vi "TestPattern.vi"() -> ()   [LabVIEW 2016]
uses:
  C:/Users/Aerotech/Documents/BNLStaveAssembly-blueprint/Bin/Aerotech.A3200.dll
  BNLStaveAssembly-blueprint/Bin/Aerotech.A3200.dll
  <vilib>/Utility/file.llb/Read Delimited Spreadsheet (DBL).vi
  <vilib>/Utility/file.llb/Write Delimited Spreadsheet (DBL).vi
  <vilib>/Utility/file.llb/Write Delimited Spreadsheet (I64).vi
panel:
  out "y length":i32
  out "x length":i32
  in  "y array":path
  out "y array":dbl[](array[numeric])
  in  "path to just x array":path
  out "just x array":dbl[](array[numeric])
  out "trial 2":cluster{dbl[], dbl[]}
  in  "Lowest Z Position":dbl=38.0
  in  "XYZ Stage Control":refnum<k24>
  in  "Axis speeds (mm/s)":T1={"vX [mm]"=49.0, "vY [mm]"=49.0, "vZ [mm] "=49.0}
  out "Final Position":T2={"Final X"=-325.49379764644783, "Final Y"=23.533617154160947, "Final Z"=34.99956596392527}
  out "y coord":dbl[](array[numeric])
  out "x coord":dbl[](array[numeric])
  out "all coords":dbl[][](array[numeric])
  in  "file path (dialog if empty)":path
  in  "append to file? (new file:F)":bool
  in  "x dist":dbl=90.0
  in  "y dist":dbl=90.0
  out "Trial 1":dbl[][](array[numeric])
  out "dx":dbl
  out "dy":dbl
  in  "module lenght y":dbl=90.0
  in  "module lenght x":dbl=90.0
  out "Array":bool[][](array[boolean])
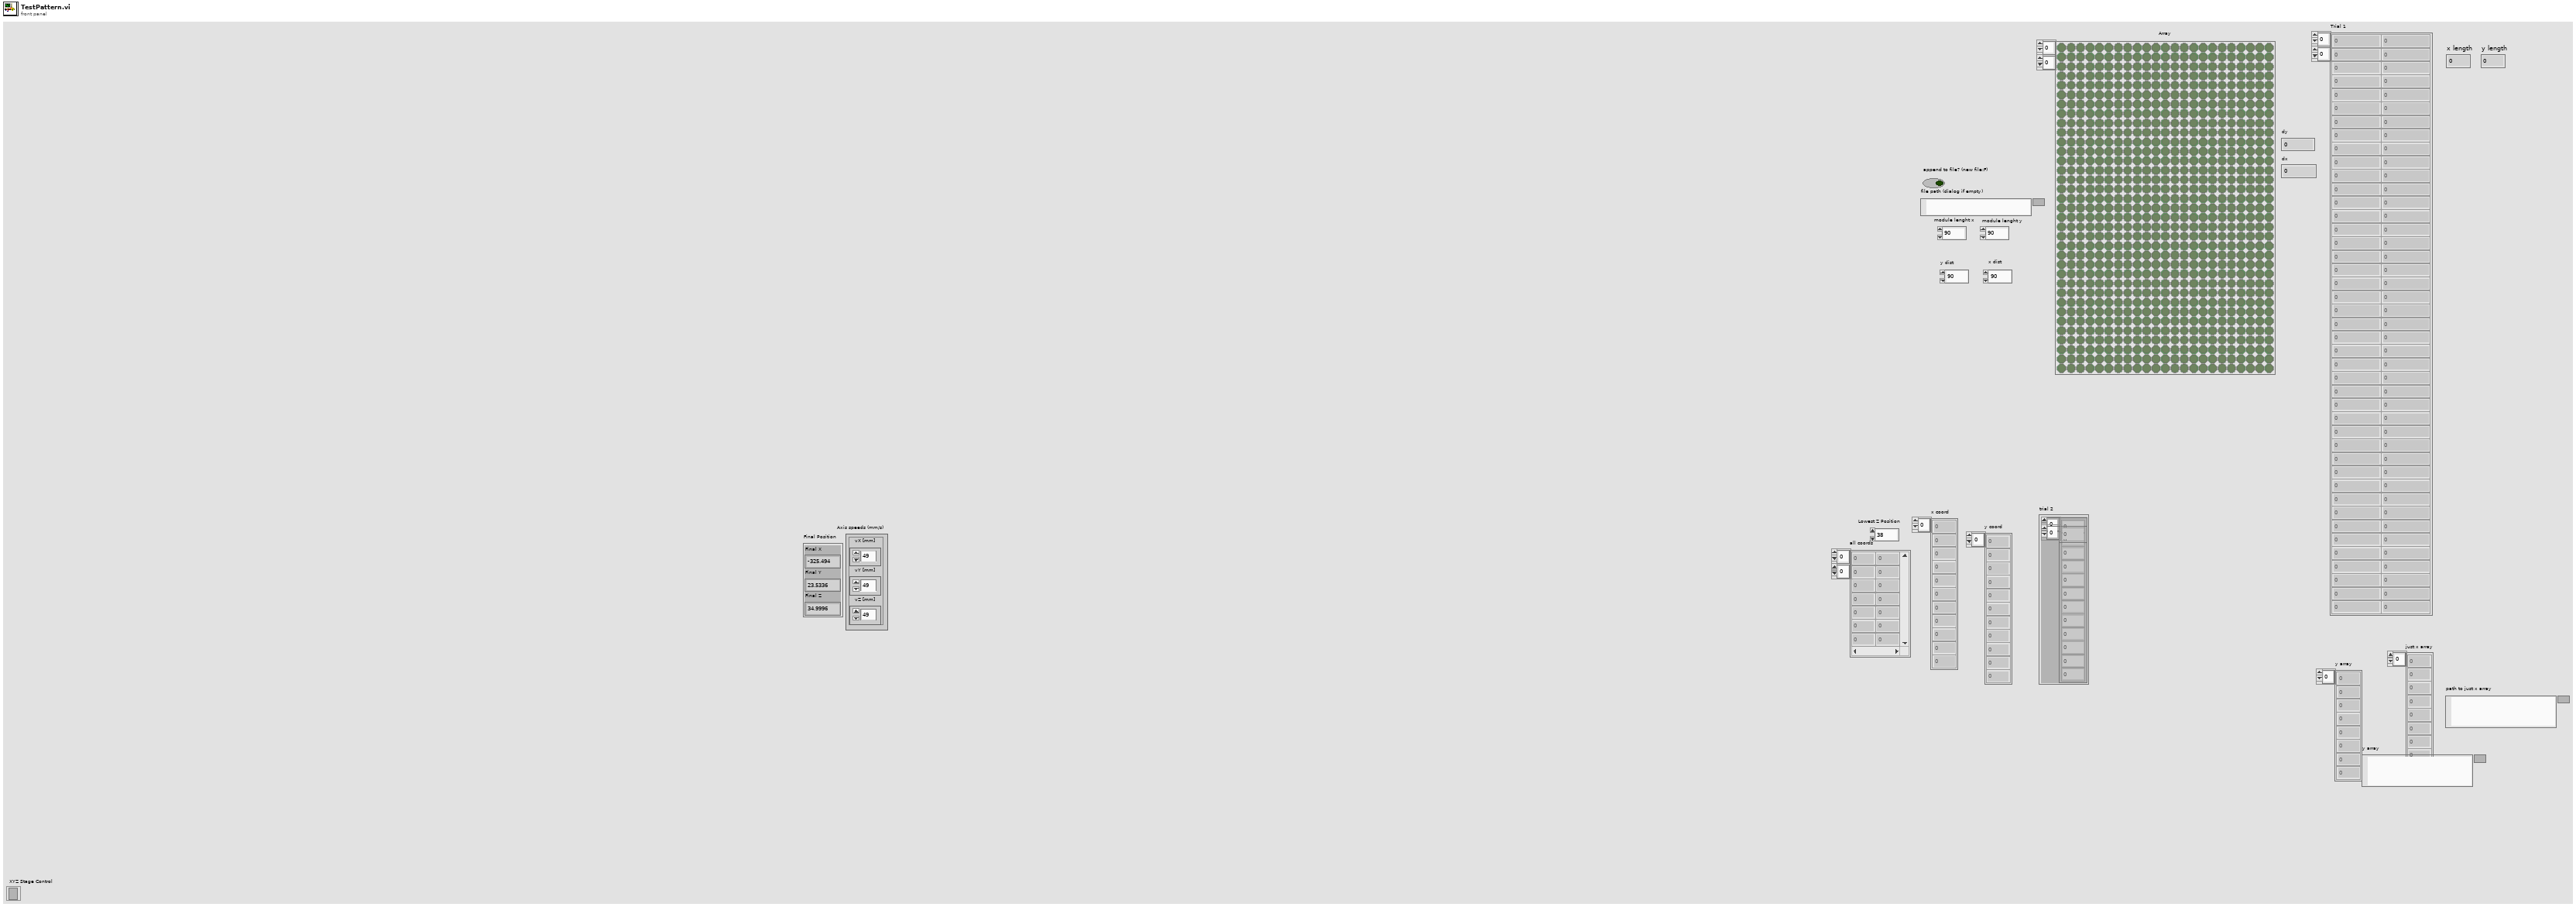
[diagram p1: front panel]
types:
  T1 = cluster{"vX [mm]":dbl, "vY [mm]":dbl, "vZ [mm] ":dbl}
  T2 = cluster{"Final X":dbl, "Final Y":dbl, "Final Z":dbl}
  T3 = cluster{"Numeric":dbl, "Numeric":dbl, "Lowest Z Position":dbl}
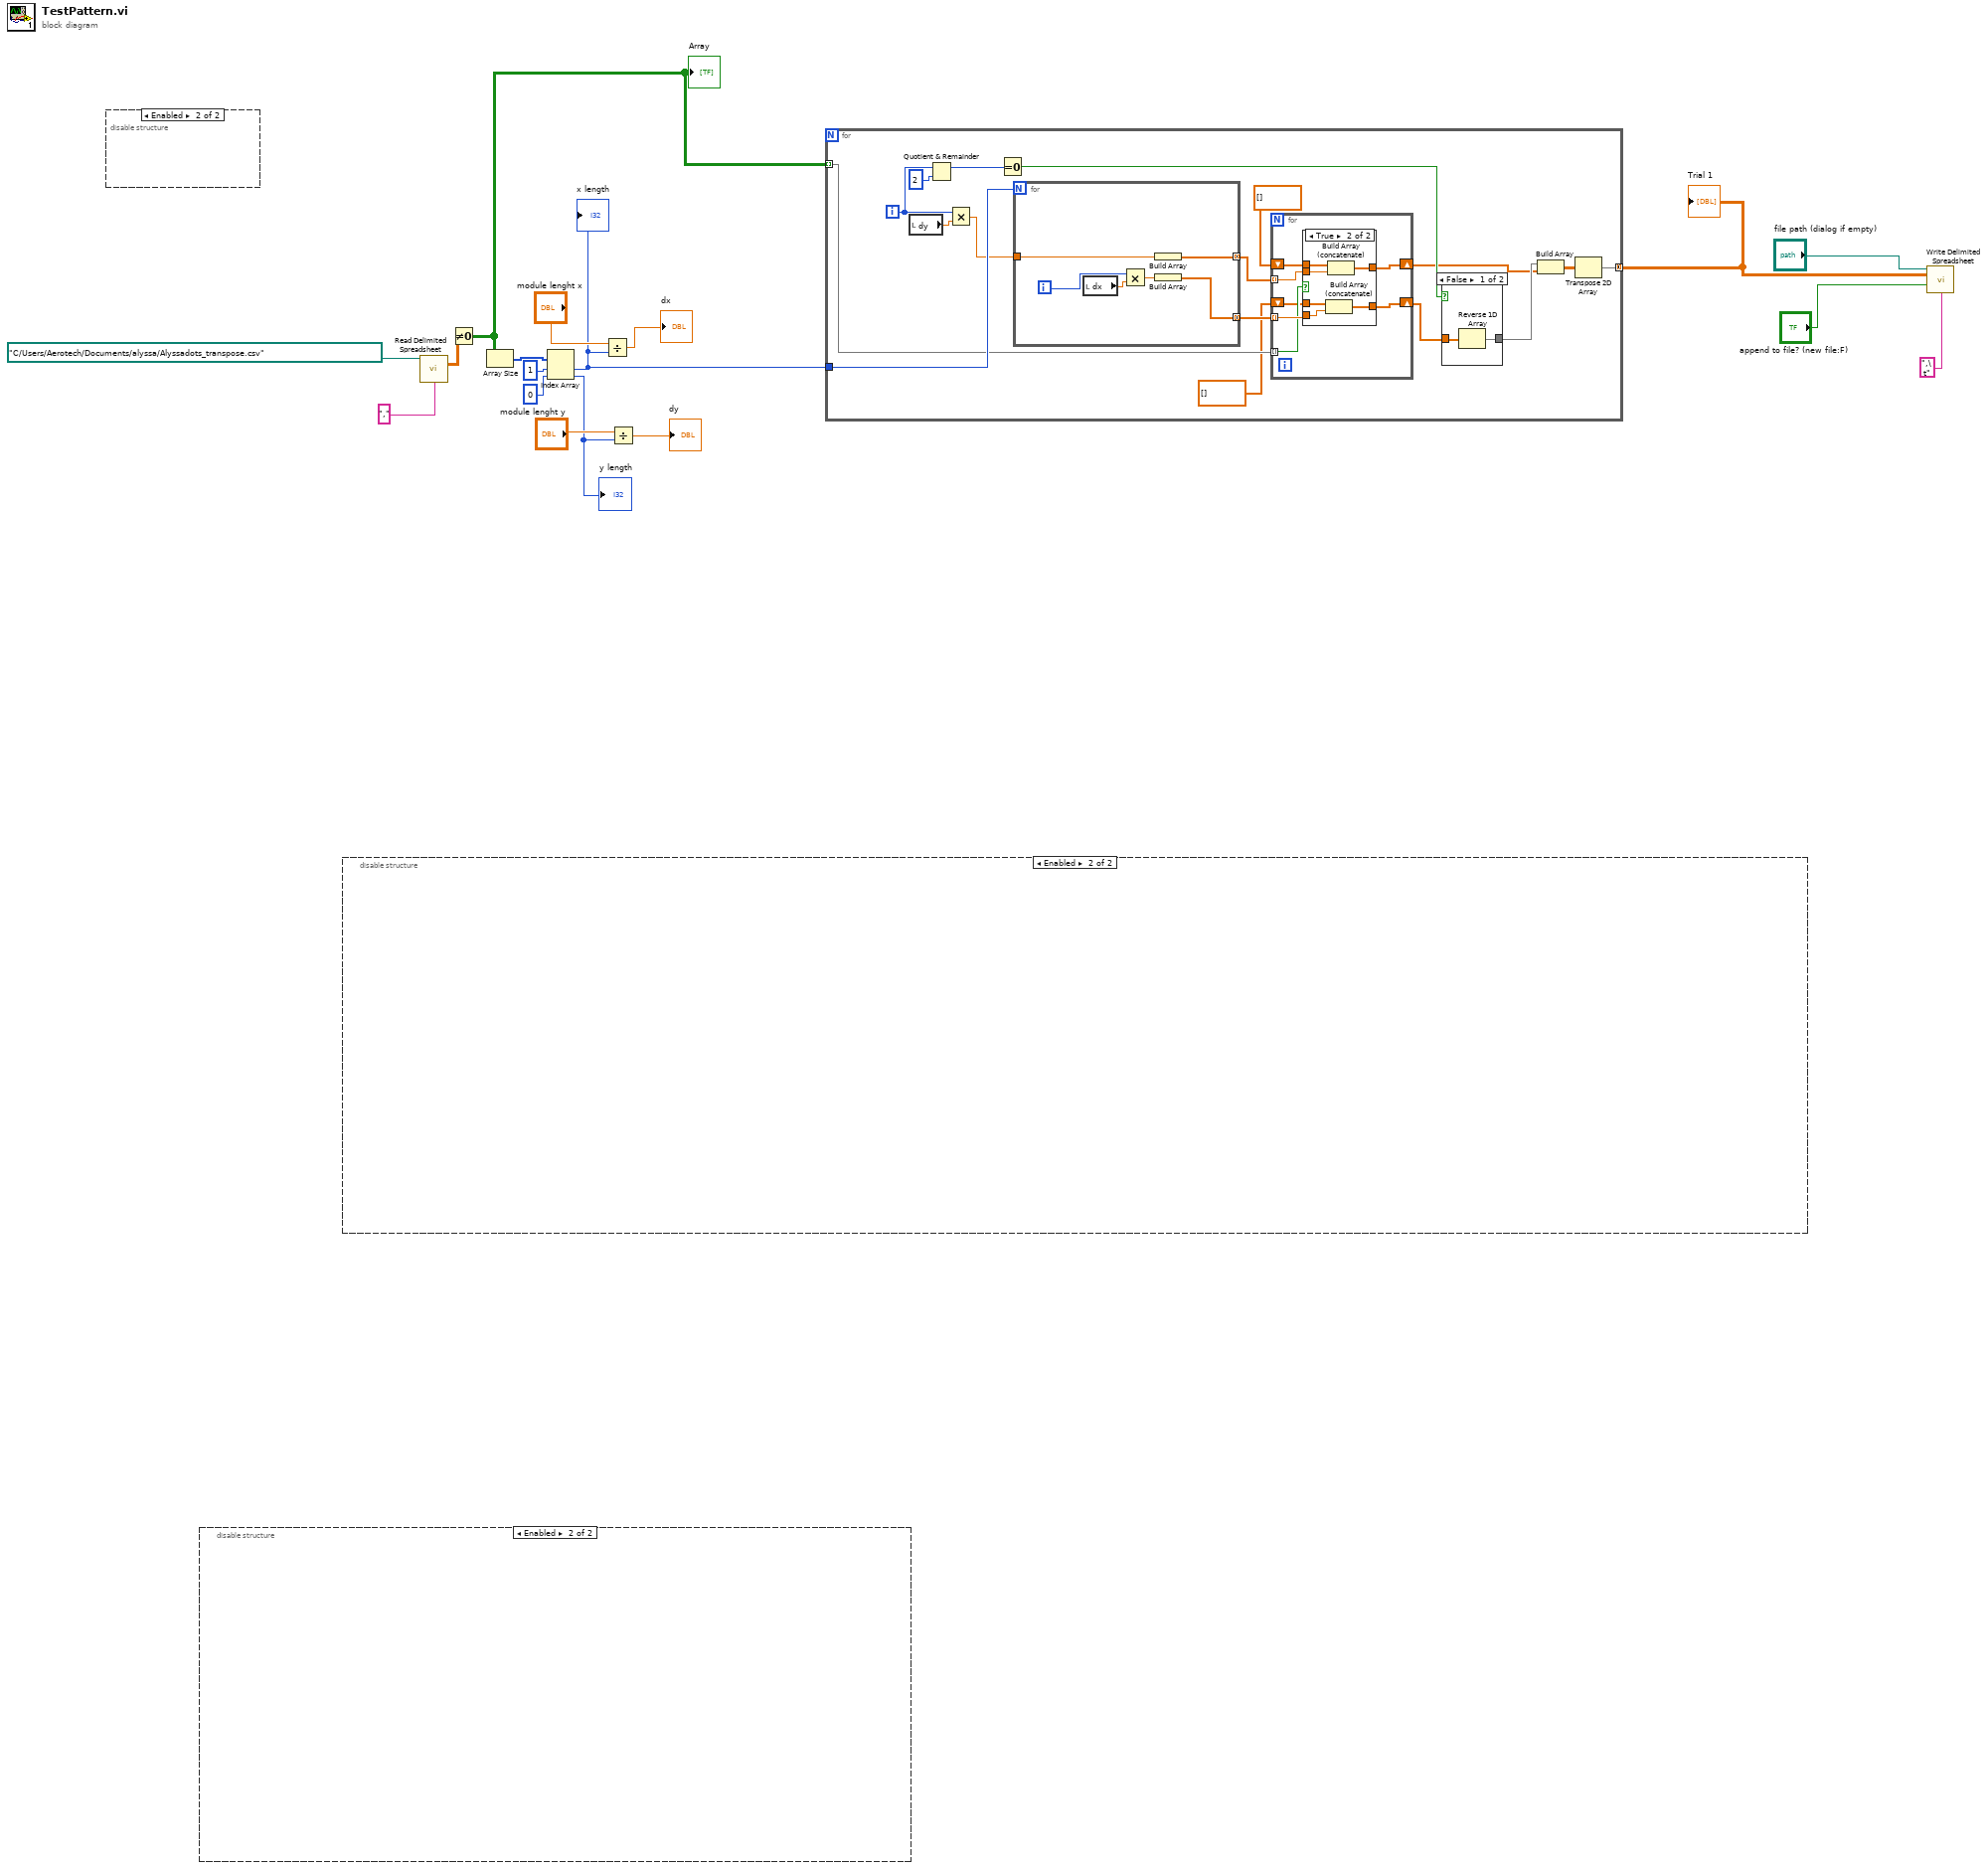
[diagram p0: block diagram]
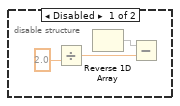
[diagram p4: hidden frame]
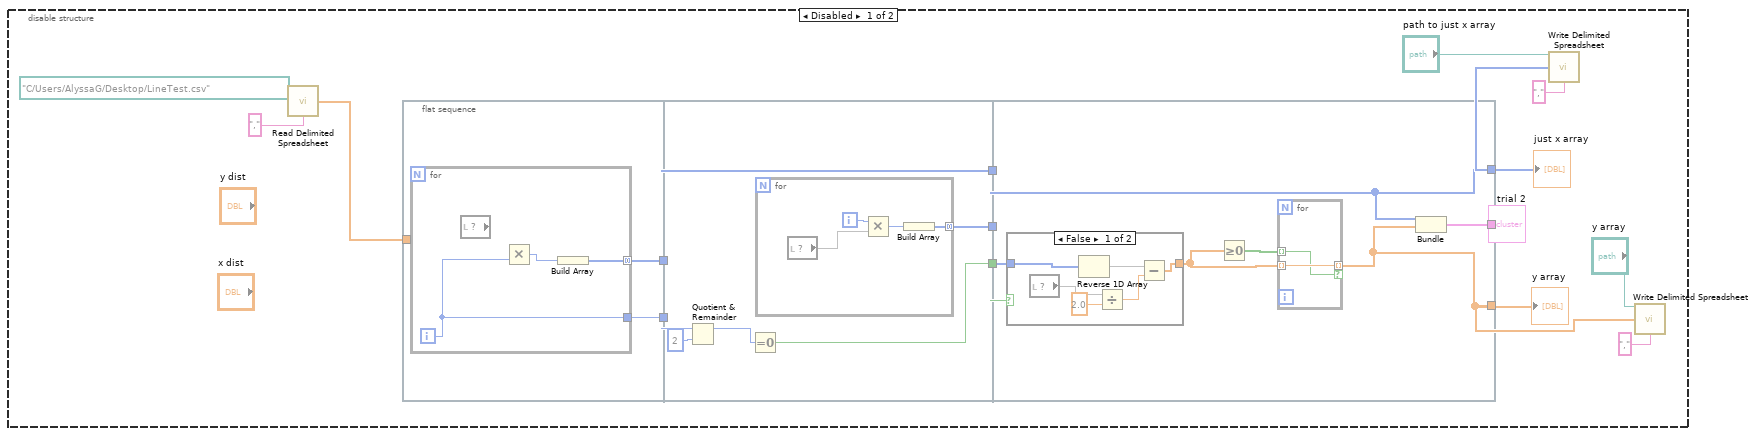
[diagram p5: hidden frame]
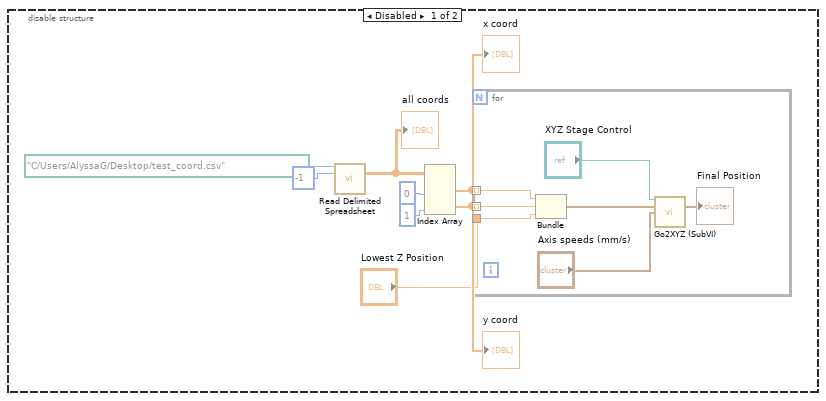
[diagram p7: hidden frame]
diagram:
  n1 = disable-structure shown="Enabled" {
    frame Disabled {
      n2 = Divide(y=2.0) -> (x/y=w19:dbl)  [unwired: 1 in]
      n3 = Reverse 1D Array() -> (reversed array=w20:dbl[])  [unwired: 1 in]
      n4 = Subtract(x=w20, y=w19) -> ()  [unwired: 1 out]
    }
    frame Enabled {
    }
  }
  n5 = disable-structure shown="Enabled" {
    frame Disabled {
      n6 = call-poly <vilib>:"Read Delimited Spreadsheet.vi"("file path (dialog if empty)"=path "C:/Users/AlyssaG/Desktop/test_coord.csv", "number of rows (all:-1)"=-1) -> ("all rows"=w26:dbl[][])  [unwired: 8 in, 5 out]
      "all coords" <- w26
      n7 = Index Array(array=w26, index (col) #1=0 ("index"), index (col) #2=1 ("index")) -> (element #1=w23:dbl[], element #2=w22:dbl[])  [unwired: 2 in]
      "x coord" <- w23
      "y coord" <- w22
      n8 = for {
        tunnel: w23 -> [w33] mode=indexing
        tunnel: w22 -> [w32] mode=indexing
        tunnel: "Lowest Z Position" -> [w31]
        n9 = Bundle("Numeric"=w33, "Numeric"=w32, "Lowest Z Position"=w31) -> (w30:T3)  [unwired: 1 in]
        n10 = call "Go2XYZ (SubVI).vi"(".NET Refnum in"="XYZ Stage Control", "Go to Coordinates"=w30, "Axis Speeds"="Axis speeds (mm/s)") -> ("Final Position"=→"Final Position":T2)  [unwired: 8 in, 4 out]
      }
    }
    frame Enabled {
    }
  }
  n11 = disable-structure shown="Enabled" {
    frame Disabled {
      n12 = call-poly <vilib>:"Read Delimited Spreadsheet.vi"("file path (dialog if empty)"=path "C:/Users/AlyssaG/Desktop/LineTest.csv", "delimiter (\\t)"="," ("delimiter (\\t)")) -> ("first row"=w36:dbl[])  [unwired: 8 in, 5 out]
      n13 = flat-sequence {
        tunnel: [w52] -> w50
        tunnel: [w51] -> w49
        tunnel: w36 -> [_]
        tunnel: [w59] -> w48
        tunnel: [w58] -> w47
        tunnel: [w57] -> w46
        tunnel: w50 -> [w57]
        tunnel: w49 -> [w56]
        tunnel: w48 -> [w71]
        tunnel: w47 -> [w72]
        tunnel: w46 -> [w67]
        tunnel: [w68] -> w45
        tunnel: [w67] -> w44
        tunnel: [w66] -> w41
        frame #0 {
          n14 = for {
            tunnel: [w54] -> w52 mode=concatenating
            tunnel: [w53] -> w51
            i -> [w53]
            n15 = local read item#-1() -> ()  [unwired: 1 out]
            n16 = Multiply(y=w53) -> (x*y=w55:i32)  [unwired: 1 in]
            n17 = Build Array(w55) -> (w54:i32[])
          }
        }
        frame #1 {
          n18 = Quotient & Remainder(x=w56, y=2) -> (x-y*floor(x/y)=w60:i32)  [unwired: 1 out]
          n19 = Equal To 0?(x=w60) -> (x = 0?=w58:bool)
          n20 = for {
            tunnel: [w62] -> w59 mode=concatenating
            i -> [w64]
            n21 = local read item#-1() -> (w65)
            n22 = Multiply(x=w64, y=w65) -> (x*y=w63:i32)
            n23 = Build Array(w63) -> (w62:i32[])
          }
        }
        frame #2 {
          n24 = case shown="False" w72 {
            tunnel: [w75 w81] -> w69
            tunnel: w71 -> [w80 w81]
            frame False {
              n25 = local read item#-1() -> (w78)
              n26 = Reverse 1D Array(array=w80) -> (reversed array=w76:i32[])
              n27 = Divide(x=w78, y=2.0) -> (x/y=w77:dbl)
              n28 = Subtract(x=w76, y=w77) -> (x-y=w75:dbl[])
            }
            frame True {
            }
          }
          n29 = Greater Or Equal To 0?(x=w69) -> (x >= 0?=w70:bool[])
          n30 = for {
            tunnel: w70 -> [w73] mode=indexing
            tunnel: w69 -> [w74] mode=indexing
            tunnel: [w74] -> w66 mode=indexing if=w73
          }
          n31 = Bundle(w67, w66) -> (w68:cluster{i32[], dbl[]})  [unwired: 1 in]
        }
      }
      n32 = call-poly <vilib>:"Write Delimited Spreadsheet.vi"("file path (dialog if empty)"="path to just x array", "1D data"=w44, "delimiter (\\t)"="," ("delimiter (\\t)")) -> ()  [unwired: 11 in, 2 out]
      n33 = call-poly <vilib>:"Write Delimited Spreadsheet.vi"("file path (dialog if empty)"="y array", "1D data"=w41, "delimiter (\\t)"="," ("delimiter (\\t)")) -> ()  [unwired: 11 in, 2 out]
      "trial 2" <- w45
      "just x array" <- w44
      "y array" <- w41
    }
    frame Enabled {
    }
  }
  n34 = call-poly <vilib>:"Read Delimited Spreadsheet.vi"("file path (dialog if empty)"=path "C:/Users/Aerotech/Documents/alyssa/Alyssadots_transpose.csv" ("file (use dialog)"), "delimiter (\\t)"="," ("delimiter (\\t)")) -> ("all rows"=w11:dbl[][])  [unwired: 8 in, 5 out]
  n35 = Not Equal To 0?(x=w11) -> (x != 0?=w4:bool[][])
  "Array" <- w4
  n36 = Array Size(array=w4) -> (size(s)=w15:i32[])
  n37 = Index Array(array=w15, index #1=1 ("index"), index #2=0 ("index")) -> (element #1=w6:i32, element #2=w5:i32)
  "x length" <- w6
  "y length" <- w5
  n38 = Divide(x="module lenght x", y=w6) -> (x/y=→"dx":dbl)
  n39 = Divide(x="module lenght y", y=w5) -> (x/y=→"dy":dbl)
  n40 = for {
    tunnel: w6 -> [w97]
    tunnel: [w96] -> w7 mode=concatenating
    tunnel: w4 -> [w88] mode=indexing
    i -> [w98]
    n41 = local read "dy"() -> (w95:dbl)
    n42 = Quotient & Remainder(x=w98, y=2) -> (x-y*floor(x/y)=w94:i32)  [unwired: 1 out]
    n43 = Multiply(x=w98, y=w95) -> (x*y=w93:dbl)
    n44 = Equal To 0?(x=w94) -> (x = 0?=w90:bool)
    n45 = for {
      N: w97 -> [_]
      tunnel: w93 -> [w121]
      tunnel: [w120] -> w87 mode=concatenating
      tunnel: [w119] -> w86 mode=concatenating
      i -> [w122]
      n46 = local read "dx"() -> (w118:dbl)
      n47 = Multiply(x=w122, y=w118) -> (x*y=w117:dbl)
      n48 = Build Array(w121) -> (w119:dbl[])
      n49 = Build Array(w117) -> (w120:dbl[])
    }
    n50 = for {
      tunnel: w87 -> [w105] mode=indexing
      tunnel: w86 -> [w99] mode=indexing
      tunnel: w88 -> [w104] mode=indexing
      shift-right: [w102] -> w84
      shift-left: dbl[] [] -> [w103]
      shift-right: [w101] -> w85
      shift-left: dbl[] [] -> [w100]
      n51 = case shown="True" w104 {
        tunnel: [w107 w113] -> w102
        tunnel: w105 -> [_ w112]
        tunnel: w99 -> [_ w108]
        tunnel: w103 -> [w107 w109]
        tunnel: [w106 w111] -> w101
        tunnel: w100 -> [w106 w110]
        frame False {
        }
        frame True {
          n52 = Build Array (concatenate)(w110, w112) -> (w111:dbl[])
          n53 = Build Array (concatenate)(w109, w108) -> (w113:dbl[])
        }
      }
    }
    n54 = case shown="False" w90 {
      tunnel: [w114 w116] -> w89
      tunnel: w85 -> [w115 w116]
      frame False {
        n55 = Reverse 1D Array(array=w115) -> (reversed array=w114:dbl[])
      }
      frame True {
      }
    }
    n56 = Build Array(w89, w84) -> (w91:dbl[][])
    n57 = Transpose 2D Array(2D array=w91) -> (transposed array=w96:dbl[][])
  }
  "Trial 1" <- w7
  n58 = call-poly <vilib>:"Write Delimited Spreadsheet.vi"("file path (dialog if empty)"="file path (dialog if empty)", "2D data"=w7, "append to file? (new file:F)"="append to file? (new file:F)", "delimiter (\\t)"=",\t" ("delimiter (\\t)")) -> ()  [unwired: 10 in, 2 out]
